vi "RC_Set_Parameters.vi"(8 "error in (no error)":errorcluster, 11 "Reward_Condition in":refnum<class "Reward_Condition.lvclass">) -> (0 "error out":errorcluster, 3 "Reward_Condition out":refnum<class "Reward_Condition.lvclass">)   [LabVIEW 2018, in "Tracker.lvlib" / "Reward_Condition.lvclass"]
uses:
  Reward_Condition.lvclass
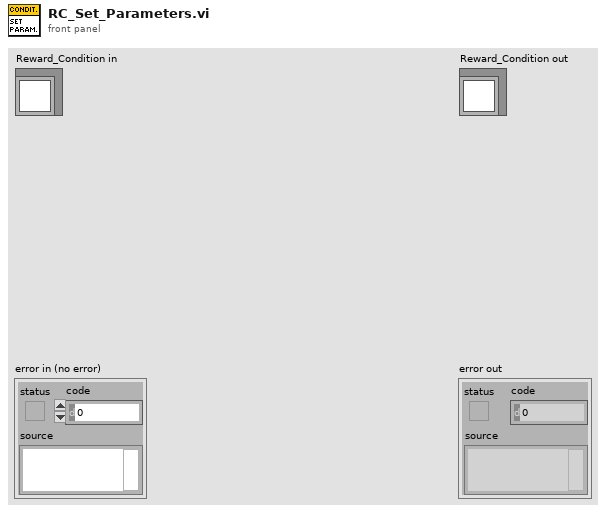
[diagram p1: front panel]
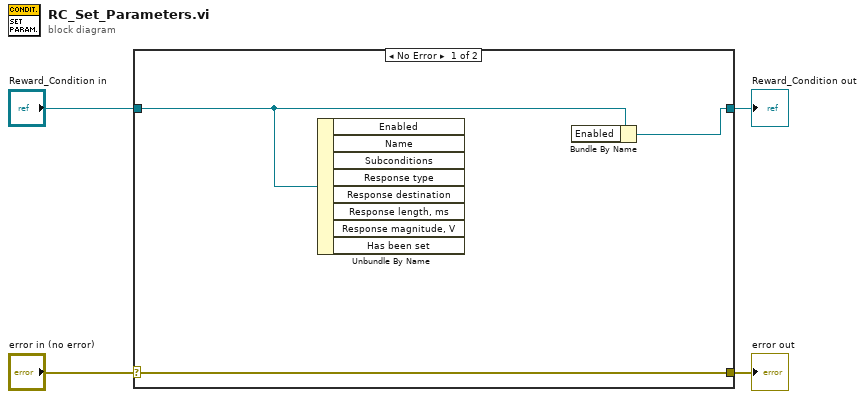
[diagram p0: block diagram]
diagram:
  n1 = case shown="No Error" "error in (no error)" {
    selector: "error in (no error)" -> [w7 w9]
    tunnel: [w7 w9] -> w3
    tunnel: [w5 w8] -> w1
    tunnel: "Reward_Condition in" -> [w6 w8]
    frame No Error {
      n2 = Unbundle By Name(w6) -> ()  [unwired: 8 out]
      n3 = Bundle By Name(cluster=w6) -> (w5:refnum<class "Reward_Condition.lvclass">)  [unwired: 1 in]
    }
    frame Error {
    }
  }
  "error out" <- w3
  "Reward_Condition out" <- w1
